vi "HEWH Agilent Create Data Array.vi"(8 "Error In":errorcluster, 9 "Agilent Calibrated Cluster Array":T1, 10 "Agilent Raw Cluster Array":T1, 11 "Data In":string[](array[string])) -> (0 "Error Out":errorcluster, 3 "Data Out":string[](array[string]))   [LabVIEW 2020]
uses:
  Type Definitions/HEWH Agilent Cluster.ctl
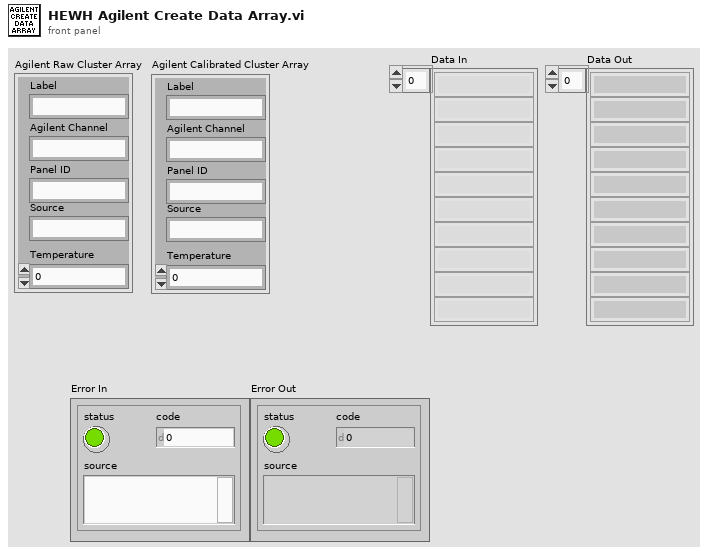
[diagram p1: front panel]
types:
  T1 = typedef "HEWH Agilent Cluster.ctl" = cluster{"Label":string, "Agilent Channel":string, "Panel ID":string, "Source":string, "Temperature":dbl}
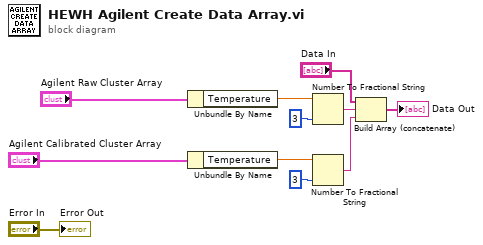
[diagram p0: block diagram]
diagram:
  n1 = Unbundle By Name("Agilent Raw Cluster Array") -> ("Temperature"=w2:dbl)
  n2 = Unbundle By Name("Agilent Calibrated Cluster Array") -> ("Temperature"=w9:dbl)
  n3 = Number To Fractional String(number=w2, precision (6)=i16 3) -> (F-format string=w7:string)  [unwired: 2 in]
  n4 = Number To Fractional String(number=w9, precision (6)=i16 3) -> (F-format string=w10:string)  [unwired: 2 in]
  n5 = Build Array (concatenate)("Data In", w7, w10) -> (→"Data Out":string[])
  "Error Out" <- "Error In"
